vi "GetOutput.vi"(6 "error in":errorcluster, 9 "Tunnel in":refnum<class "Tunnel.lvclass">) -> (0 "error out":errorcluster, 3 "Tunnel out":refnum<class "Tunnel.lvclass">, 4 "name":string)   [LabVIEW 2014, in "Tunnel.lvclass"]
uses:
  Tunnel.lvclass
  Tunnel.lvclass/Tunnel.ctl
  Terminal/Terminal.lvclass
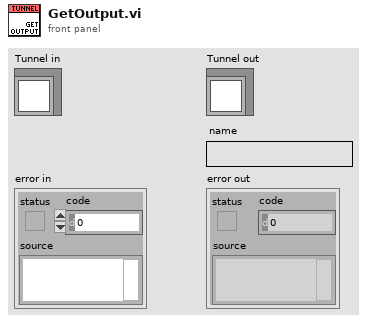
[diagram p1: front panel]
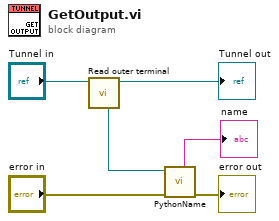
[diagram p0: block diagram]
diagram:
  n1 = call "Read outer terminal.vi"("Tunnel in"="Tunnel in") -> ("Tunnel out"=→"Tunnel out":refnum<class "Tunnel.lvclass">, "outer terminal"=w4:refnum<class "Terminal.lvclass">)  [unwired: 7 in]
  n2 = call-dynamic "PythonName.vi"("error in"="error in", "Terminal in"=w4) -> ("error out"=→"error out":errorcluster, "name"=→"name":string)  [unwired: 6 in, 2 out]
